vi "GetLEDColour.vi"(11 "Command status":string="UNDEF") -> (3 "Colors [4]":cluster{u32, u32}[](array[cluster]))   [LabVIEW 2012, in "ValveController.lvlib"]
uses:
  <instrlib>/ValveController/ValveController.lvlib
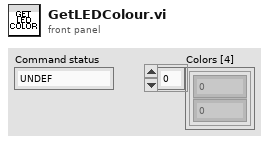
[diagram p1: front panel]
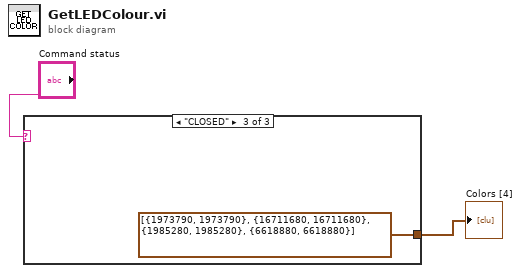
[diagram p0: block diagram]
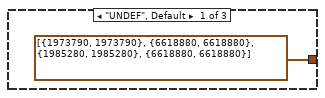
[diagram p2: hidden frame]
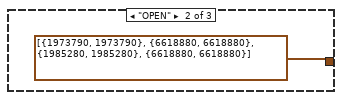
[diagram p3: hidden frame]
diagram:
  n1 = case shown="\"CLOSED\"" "Command status" {
    tunnel: [cluster{u32, u32}[] [{1973790, 1973790}, {6618880, 6618880}, {1985280, 1985280}, {6618880, 6618880}] ("Colors [4]") cluster{u32, u32}[] [{1973790, 1973790}, {6618880, 6618880}, {1985280, 1985280}, {6618880, 6618880}] ("Colors [4]") cluster{u32, u32}[] [{1973790, 1973790}, {16711680, 16711680}, {1985280, 1985280}, {6618880, 6618880}] ("Colors [4]")] -> w2
    frame "UNDEF", Default {
    }
    frame "OPEN" {
    }
    frame "CLOSED" {
    }
  }
  "Colors [4]" <- w2
